vi "Frame Page.vi"(8 "error in (no error)":errorcluster, 11 "Node Ptr":T2 format="%.0x") -> (0 "error out":errorcluster)   [LabVIEW 2015, in "J1939 Addon System Explorer.lvlib"]
uses:
  J1939 Addon System Explorer.lvlib
  <vilib>/NI Veristand/Custom Device API/Custom Device Item Ref.ctl
  NationalInstruments.VeriStand.SystemStorageUI
  Shared/Types/Outgoing Event Trigger Types.ctl
  <vilib>/NI Veristand/UI Controls/Single Node Browser/Net Event Data.ctl
  <vilib>/NI Veristand/UI Controls/Single Node Browser/Net Event.ctl
  Shared/J1939 Utilities/SubVIs/Convert CAN Arb ID to J1939 ID.vi
  Shared/SubVIs/Constants.vi
  <vilib>/NI VeriStand/Custom Device API/Custom Device API.lvlib
  Shared/J1939 Utilities/J1939 Utilities.lvlib
  Shared/J1939 Addon Shared.lvlib
  <vilib>/NI Veristand/UI Controls/Single Node Browser/NI_VS UI Single Node Browser.lvlib
panel:
  in  "Transmit Trigger":T1
  in  "Trigger":refnum<k24>(container)
  in  "Trigger Settings":cluster{"Section Name":string}={"Section Name"="Transmission Trigger"}
  in  "Trigger":refnum<k24>(container)
  in  "Disable Transmission":bool
  in  "Disable Settings":cluster{"Section Name":string}={"Section Name"="Disable Transmission"}
  in  "Description":string
  out "Source Address":u8 format="%.0x"
  out "Priority":u8 format="%.0x"
  out "PGN":u32 format="%.0x"
  out "Frame ID":u32 format="%.0x"
  in  "Custom Device Settings":cluster{"Section Name":string}={"Section Name"="Custom Device Item Settings"}
  out "Name":string
  in  "SHDocVw.IWebBrowser2":refnum<k7>(container)
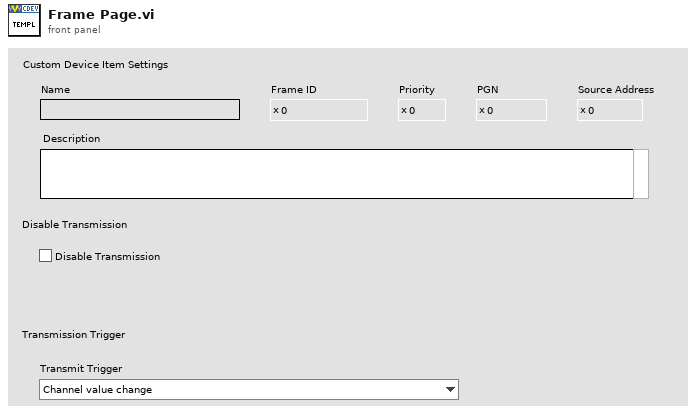
[diagram p1: front panel]
types:
  T1 = typedef "J1939 Addon Shared.lvlib/Outgoing Event Trigger Types.ctl" = enum16{"Channel value change", "Trigger channel (not zero)", "Channel value change or trigger channel (not zero)", "Trigger channel (any value change)", "Channel value change or trigger channel (any value change)"}
  T2 = typedef "Custom Device API.lvlib/Custom Device Item Ref.ctl" = u64
  T3 = cluster{"Trigger":refnum<user-event>, "Transmission":refnum<user-event>}
  T4 = typedef "J1939 Addon System Explorer.lvlib/Frame.Settings.ctl" = cluster{"ID":u32, "Disable Transmission":bool, "Disable Transmission Ref":T2, "Transmit Trigger":T1, "Transmit Trigger Ref":T2}
  T5 = typedef "Custom Device API.lvlib/Custom Device Item Info.ctl" = cluster{"Name":string, "Is Channel":bool, "GUID":string, "Is Waveform":bool}
  T6 = typedef "NI_VS UI Single Node Browser.lvlib/Single Node Browser Ref.ctl" = refnum<k24>
  T7 = typedef "NI_VS UI Single Node Browser.lvlib/Callback Type.ctl" = cluster{"Net Callbacks":refnum<k27>[], "Event":refnum<user-event>}
  T8 = typedef "Custom Device API.lvlib/Custom Device Commands.ctl" = enum16{"Default", "Item renamed", "Shutdown", "Dynamic button pressed"}
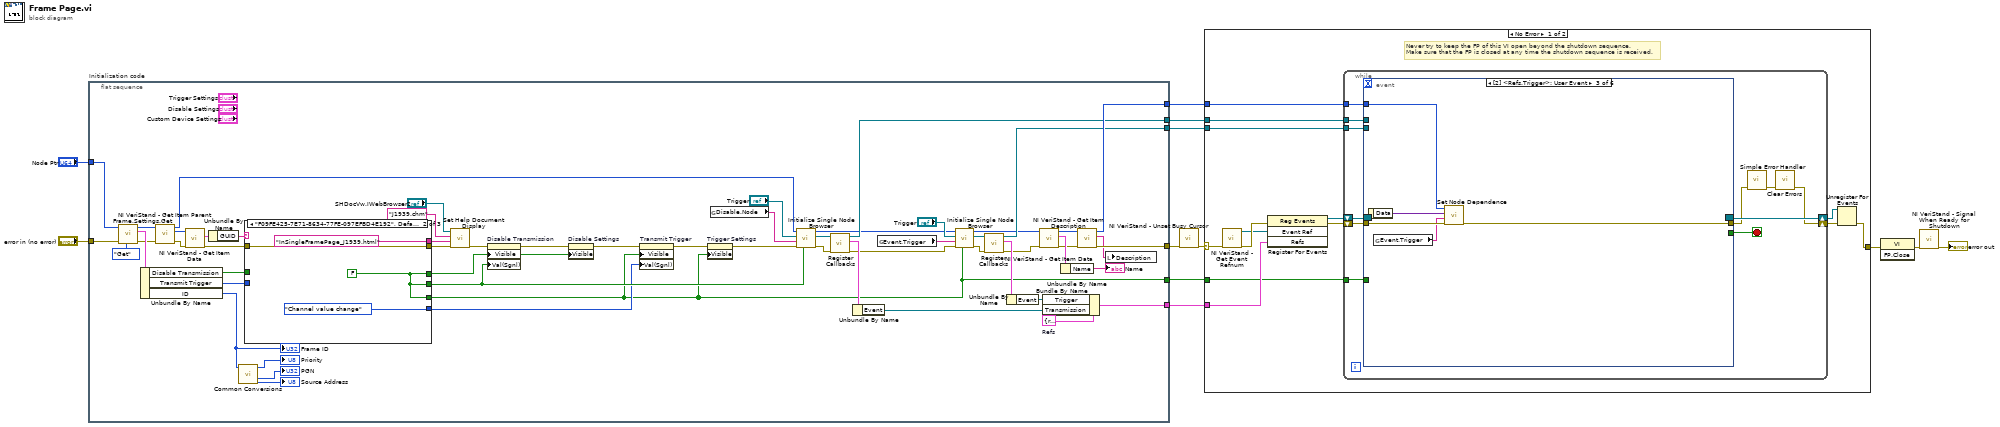
[diagram p0: block diagram]
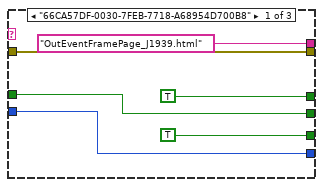
[diagram p2: hidden frame]
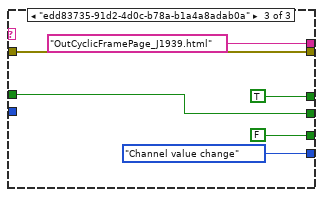
[diagram p3: hidden frame]
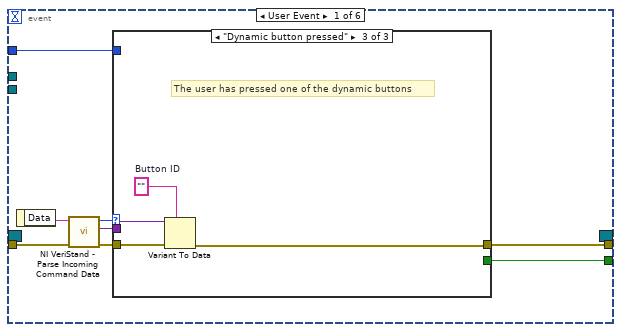
[diagram p4: hidden frame]
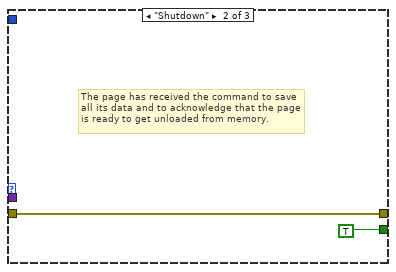
[diagram p6: hidden frame]
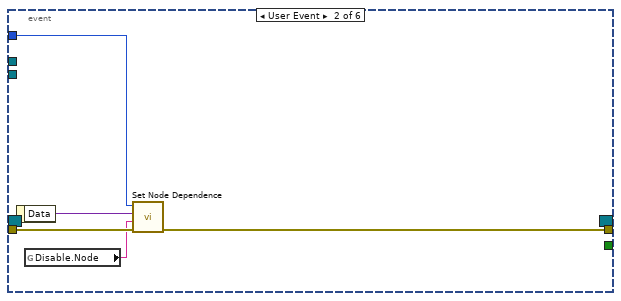
[diagram p7: hidden frame]
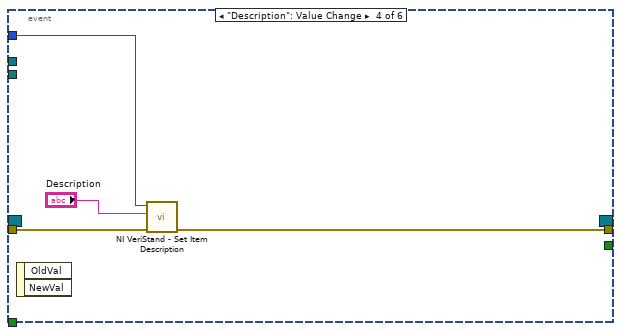
[diagram p8: hidden frame]
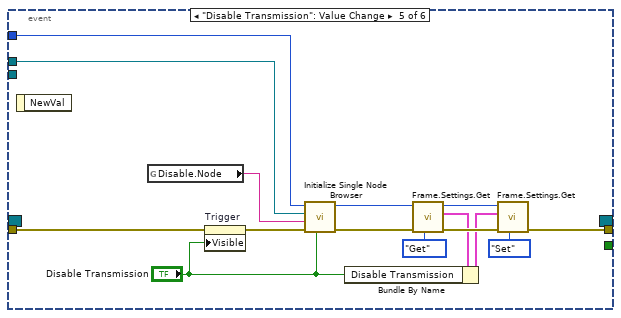
[diagram p9: hidden frame]
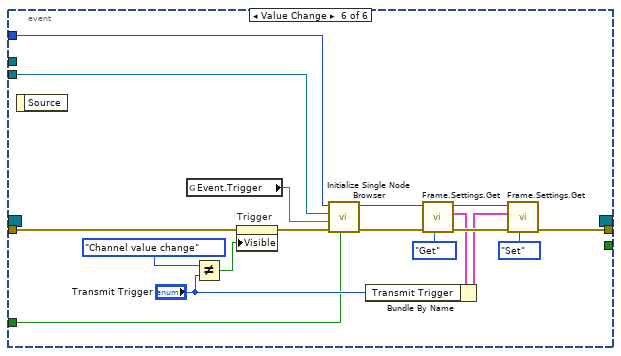
[diagram p10: hidden frame]
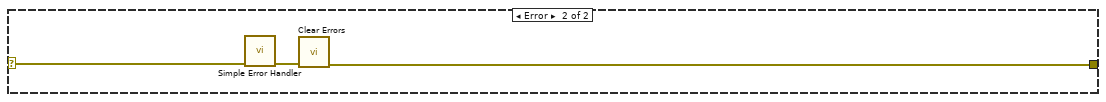
[diagram p11: hidden frame]
diagram:
  n1 = flat-sequence "Initialization code" {
    tunnel: "error in (no error)" -> [w20]
    tunnel: "Node Ptr" -> [w18]
    tunnel: [w61] -> w7
    tunnel: [w59] -> w5
    tunnel: [w42] -> w4
    tunnel: [w45] -> w3
    tunnel: [w33] -> w2
    tunnel: [w13] -> w1
    frame #0 {
      w37 = T3 {"Trigger"=refnum, "Transmission"=refnum}  # Refs
      n2 = call "Frame.Settings.Get.vi"("Action"=enum8{"Get", "Set"}."Get", "error in (no error)"=w20, "Item Ref in"=w18) -> ("error out"=w19:errorcluster, "Frame.Settings"=w24:T4, "Item Ref out"=w17:T2)  [unwired: 6 in]
      n3 = Unbundle By Name(w24) -> ("Disable Transmission"=w16:bool, "Transmit Trigger"=w15:T1, "ID"=w23:u32)
      "Frame ID" <- w23
      n4 = call <vilib>:"NI VeriStand - Get Item Parent.vi"("error in (no error)"=w19, "Item Ref in"=w17) -> ("error out"=w57:errorcluster, "Parent Ref"=w56:T2, "Item Ref out"=w49:T2)  [unwired: 6 in, 1 out]
      n5 = call <vilib>:"NI VeriStand - Get Item Data.vi"("error in (no error)"=w57, "Item Ref in"=w56) -> ("error out"=w53:errorcluster, "Item Info"=w55:T5)  [unwired: 8 out]
      n6 = Unbundle By Name(w55) -> ("GUID"=w54:string)
      n7 = call-poly "Common Conversions.vi"("Arb ID"=w23) -> ("Priority"=→"Priority":u8, "PGN"=→"PGN":u32, "Source Address"=→"Source Address":u8)  [unwired: 11 in, 1 out]
      n8 = case shown="\"F09FE425-7E71-8634-77FE-097EFBD4E192\", Default" w54 {
        tunnel: ["OutEventFramePage_J1939.html" ("HTML File") "InSingleFramePage_J1939.html" ("HTML File") "OutCyclicFramePage_J1939.html" ("HTML File")] -> w69
        tunnel: w53 -> [w75 w79 w85]
        tunnel: [w75 w79 w85] -> w26
        tunnel: [TRUE w78 TRUE] -> w46
        tunnel: [w71 w78 w82] -> w28
        tunnel: [TRUE w78 FALSE] -> w13
        tunnel: [w72 Outgoing_Event_Trigger_Types."Channel value change" ("y") Outgoing_Event_Trigger_Types."Channel value change" ("y")] -> w27
        tunnel: w16 -> [w71 _ w82]
        tunnel: w15 -> [w72 _ _]
        frame "66CA57DF-0030-7FEB-7718-A68954D700B8" {
        }
        frame "F09FE425-7E71-8634-77FE-097EFBD4E192", Default {
          w78 = FALSE
        }
        frame "edd83735-91d2-4d0c-b78a-b1a4a8adab0a" {
        }
      }
      n9 = call "Set Help Document Display.vi"("error in (no error)"=w26, "HTML File"=w69, "Main CHM File"="J1939.chm", "SHDocVw.IWebBrowser2"="SHDocVw.IWebBrowser2") -> ("error out"=w25:errorcluster)  [unwired: 7 in]
      n10 = property on="Disable Transmission" class="Bool (strict)"(error in=w25, "Visible"=w46, "Val(Sgnl)"=w28) -> (error out=w52:errorcluster)  [unwired: 1 in, 1 out]
      n11 = property on="Disable Settings" class="Clust (strict)"(error in=w52, "Visible"=w46) -> (error out=w30:errorcluster)  [unwired: 1 in, 1 out]
      n12 = property on="Transmit Trigger" class="Enum (strict)"(error in=w30, "Visible"=w13, "Val(Sgnl)"=w27) -> (error out=w29:errorcluster)  [unwired: 1 in, 1 out]
      n13 = property on="Trigger Settings" class="Clust (strict)"(error in=w29, "Visible"=w13) -> (error out=w31:errorcluster)  [unwired: 1 in, 1 out]
      n14 = global read "Constants.vi" "Disable.Node"() -> (w44:string)
      n15 = call "Initialize Single Node Browser.vi"("Use Channel?"=w28, "error in (no error)"=w31, "NodeName"=w44, "Browser Ref 2"="Trigger", "Item Ref in"=w49) -> ("error out"=w51:errorcluster, "Browser Ref"=w50:T6, "Item Ref out"=w32:T2)  [unwired: 4 in]
      n16 = call <vilib>:"Register Callbacks.vi"("error in (no error)"=w51, "Single Node Browser"=w50) -> ("error out"=w38:errorcluster, "Callbacks"=w48:T7, "Single Node Browser dup"=w45:T6)  [unwired: 7 in]
      n17 = Unbundle By Name(w48) -> ("Event"=w43:refnum<user-event>)
      n18 = global read "Constants.vi" "Event.Trigger"() -> (w35:string)
      n19 = call "Initialize Single Node Browser.vi"("Use Channel?"=w13, "error in (no error)"=w38, "NodeName"=w35, "Browser Ref 2"="Trigger", "Item Ref in"=w32) -> ("error out"=w39:errorcluster, "Browser Ref"=w40:T6, "Item Ref out"=w21:T2)  [unwired: 4 in]
      n20 = call <vilib>:"Register Callbacks.vi"("error in (no error)"=w39, "Single Node Browser"=w40) -> ("error out"=w22:errorcluster, "Callbacks"=w41:T7, "Single Node Browser dup"=w33:T6)  [unwired: 7 in]
      n21 = Unbundle By Name(w41) -> ("Event"=w36:refnum<user-event>)
      n22 = call <vilib>:"NI VeriStand - Get Item Data.vi"("error in (no error)"=w22, "Item Ref in"=w21) -> ("error out"=w62:errorcluster, "Item Info"=w67:T5, "Item Ref out"=w60:T2)  [unwired: 7 out]
      n23 = Bundle By Name(cluster=w37, "Trigger"=w36, "Transmission"=w43) -> (w42:T3)
      n24 = Unbundle By Name(w67) -> ("Name"=→"Name":string)
      n25 = call <vilib>:"NI VeriStand - Get Item Description.vi"("error in (no error)"=w62, "Item Ref in"=w60) -> ("error out"=w61:errorcluster, "Description"=w58:string, "Item Ref out"=w59:T2)  [unwired: 7 out]
      n26 = local write "Description"(w58) -> ()
    }
  }
  n27 = call <vilib>:"NI VeriStand - Unset Busy Cursor.vi"("error in (no error)"=w7) -> ("error out"=w9:errorcluster)  [unwired: 10 out]
  n28 = case shown="No Error" w9 {
    selector: w9 -> [w91 w175]
    tunnel: [w96 w173] -> w12
    tunnel: w5 -> [w92 _]
    tunnel: w4 -> [w90 _]
    tunnel: w3 -> [w89 _]
    tunnel: w2 -> [w88 _]
    tunnel: w1 -> [w87 _]
    frame No Error {
      # "Never try to keep the FP of this VI open beyond the shutdown sequence.\nMake sure that the FP is closed at any time the shutdown sequence is received."
      n29 = call <vilib>:"NI VeriStand - Get Event Refnum.vi"("error in (no error)"=w91) -> ("error out"=w99:errorcluster, "Event Ref"=w95:refnum<user-event>)  [unwired: 9 out]
      n30 = register-events(error in=w99, w95, w90) -> (reference out=w93:refnum<event-registration>, error out=w94:errorcluster)  [unwired: 1 in]
      n31 = while {
        tunnel: w92 -> [w106]
        shift-right: [w103] -> w97
        shift-left: w94 -> [w109]
        shift-right: [w110] -> w98
        shift-left: w93 -> [w108]
        tunnel: w89 -> [w102]
        tunnel: w88 -> [w101]
        tunnel: w87 -> [w100]
        stop <- w107 stop-if-true
        n32 = event shown="[2] <Refs.Trigger>: User Event" {
          selector: w108 -> [_ _ _ _ _ _]
          dyn-events: [_ _ _ _ _ _] -> w110
          timeout: _ -> [_ _ _ _ _ _]
          tunnel: w109 -> [w118 w128 w133 w139 w154 w172]
          tunnel: [w114 _ _ _ _ _] -> w107
          tunnel: [w113 w127 w132 w138 w144 w157] -> w105
          tunnel: w106 -> [w112 w129 w134 w137 w152 w171]
          tunnel: w102 -> [_ _ _ _ w153 _]
          tunnel: w101 -> [_ _ _ _ _ w166]
          tunnel: w100 -> [_ _ _ _ _ w155]
          event User Event {
            n33 = event-data() -> ("Data"=w117:string)  [unwired: 1 out]
            n34 = call <vilib>:"NI VeriStand - Parse Incoming Command Data.vi"("error in (no error)"=w118, "Incoming data"=w117) -> ("error out"=w116:errorcluster, "Outgoing data"=w111:variant, "Action"=w115:T8)  [unwired: 7 out]
            n35 = case shown="\"Dynamic button pressed\"" w115 {
              tunnel: w116 -> [w119 w120 w125]
              tunnel: [_ TRUE _] -> w114
              tunnel: [w119 w120 w122] -> w113
              tunnel: w112 -> [_ _ _]
              tunnel: w111 -> [_ _ w124]
              frame "Default", Default {
              }
              frame "Shutdown" {
                # "The page has received the command to save all its data and to acknowledge that the page is ready to get unloaded from memory."
              }
              frame "Dynamic button pressed" {
                w123 = ""  # Button ID
                # "The user has pressed one of the dynamic buttons"
                n36 = Variant To Data(error in=w125, type=w123, Variant=w124) -> (error out=w122:errorcluster)  [unwired: 1 out]
              }
            }
          }
          event User Event {
            n37 = event-data() -> ("Data"=w130:variant)  [unwired: 1 out]
            n38 = global read "Constants.vi" "Disable.Node"() -> (w126:string)
            n39 = call "Set Node Dependence.vi"("error in (no error)"=w128, "NodeName"=w126, "Data"=w130, "Item Ref in"=w129) -> ("error out"=w127:errorcluster)  [unwired: 6 in, 1 out]
          }
          event User Event {
            n40 = event-data() -> ("Data"=w135:variant)  [unwired: 1 out]
            n41 = global read "Constants.vi" "Event.Trigger"() -> (w131:string)
            n42 = call "Set Node Dependence.vi"("error in (no error)"=w133, "NodeName"=w131, "Data"=w135, "Item Ref in"=w134) -> ("error out"=w132:errorcluster)  [unwired: 6 in, 1 out]
          }
          event "Description": Value Change {
            n43 = event-data() -> ()  [unwired: 3 out]
            n44 = call <vilib>:"NI VeriStand - Set Item Description.vi"("error in (no error)"=w139, "Description"="Description", "Item Ref in"=w137) -> ("error out"=w138:errorcluster)  [unwired: 8 out]
          }
          event "Disable Transmission": Value Change {
            n45 = event-data() -> ()  [unwired: 2 out]
            n46 = global read "Constants.vi" "Disable.Node"() -> (w150:string)
            n47 = property on="Trigger" class="AXCont"(error in=w154, "Visible"="Disable Transmission") -> (error out=w151:errorcluster)  [unwired: 1 in, 1 out]
            n48 = call "Initialize Single Node Browser.vi"("Use Channel?"="Disable Transmission", "error in (no error)"=w151, "NodeName"=w150, "Browser Ref 2"=w153, "Item Ref in"=w152) -> ("error out"=w147:errorcluster, "Item Ref out"=w148:T2)  [unwired: 4 in, 1 out]
            n49 = call "Frame.Settings.Get.vi"("Action"=enum8{"Get", "Set"}."Get", "error in (no error)"=w147, "Item Ref in"=w148) -> ("error out"=w145:errorcluster, "Frame.Settings"=w142:T4, "Item Ref out"=w143:T2)  [unwired: 6 in]
            n50 = Bundle By Name(cluster=w142, "Disable Transmission"="Disable Transmission") -> (w141:T4)
            n51 = call "Frame.Settings.Get.vi"("Action"=enum8{"Get", "Set"}."Set", "error in (no error)"=w145, "Frame.Settings"=w141, "Item Ref in"=w143) -> ("error out"=w144:errorcluster)  [unwired: 5 in, 2 out]
          }
          event Value Change {
            n52 = event-data() -> ()  [unwired: 2 out]
            n53 = global read "Constants.vi" "Event.Trigger"() -> (w169:string)
            n54 = Not Equal?(x=Outgoing_Event_Trigger_Types."Channel value change" ("y"), y="Transmit Trigger") -> (x != y?=w167:bool)
            n55 = property on="Trigger" class="AXCont"(error in=w172, "Visible"=w167) -> (error out=w170:errorcluster)  [unwired: 1 in, 1 out]
            n56 = call "Initialize Single Node Browser.vi"("Use Channel?"=w155, "error in (no error)"=w170, "NodeName"=w169, "Browser Ref 2"=w166, "Item Ref in"=w171) -> ("error out"=w158:errorcluster, "Item Ref out"=w156:T2)  [unwired: 4 in, 1 out]
            n57 = call "Frame.Settings.Get.vi"("Action"=enum8{"Get", "Set"}."Get", "error in (no error)"=w158, "Item Ref in"=w156) -> ("error out"=w163:errorcluster, "Frame.Settings"=w161:T4, "Item Ref out"=w162:T2)  [unwired: 6 in]
            n58 = Bundle By Name(cluster=w161, "Transmit Trigger"="Transmit Trigger") -> (w160:T4)
            n59 = call "Frame.Settings.Get.vi"("Action"=enum8{"Get", "Set"}."Set", "error in (no error)"=w163, "Frame.Settings"=w160, "Item Ref in"=w162) -> ("error out"=w157:errorcluster)  [unwired: 5 in, 2 out]
          }
        }
        n60 = call <vilib>:"Simple Error Handler.vi"("error in (no error)"=w105) -> ("error out"=w104:errorcluster)  [unwired: 1 in, 7 out]
        n61 = call <vilib>:"Clear Errors.vi"("error in (no error)"=w104) -> ("error out"=w103:errorcluster)  [unwired: 1 in, 5 out]
      }
      n62 = Unregister For Events(event registration refnum=w98, error in=w97) -> (error out=w96:errorcluster)
    }
    frame Error {
      n63 = call <vilib>:"Simple Error Handler.vi"("error in (no error)"=w175) -> ("error out"=w174:errorcluster)  [unwired: 1 in, 7 out]
      n64 = call <vilib>:"Clear Errors.vi"("error in (no error)"=w174) -> ("error out"=w173:errorcluster)  [unwired: 1 in, 5 out]
    }
  }
  n65 = invoke class="VI" method="FP.Close"(error in=w12) -> (error out=w11:errorcluster)  [unwired: 2 in, 2 out]
  n66 = call <vilib>:"NI VeriStand - Signal When Ready for Shutdown.vi"("error in (no error)"=w11) -> ("error out"=→"error out":errorcluster)  [unwired: 10 out]
